vi "GetProgramName.vi"(8 "error in":errorcluster, 11 "VISA resource name":refnum<visa-resource-name>) -> (0 "error out":errorcluster, 2 "Currently loaded program name response":string, 3 "VISA resource name out":refnum<visa-resource-name>)   [LabVIEW 2023, in "Thermotron 8800.lvlib"]
doc: "PNAM\nCommand name: Send program name\nCommand type: Program status\nDescription: Queries the 8800 for the name of the currently loaded program. The 8800 responds with the program’s assigned name (a string up to 15 characters long). If there is no currently loaded program name available, the 8800 will respond with “Untitled”.\nSyntax: PNAM?\nData type: String\nQuery example 1: PNAM?\n8800 response: STRESS SCREEN40 (The name of the currently loaded program is STRESS SCREEN40.)\nQuery example 2: PNAM?\n8800 response: Untitled (There is no currently loaded program name available.)"
uses:
  Thermotron 8800.lvlib
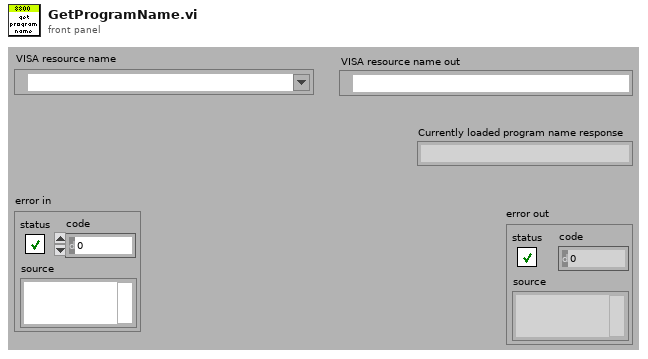
[diagram p1: front panel]
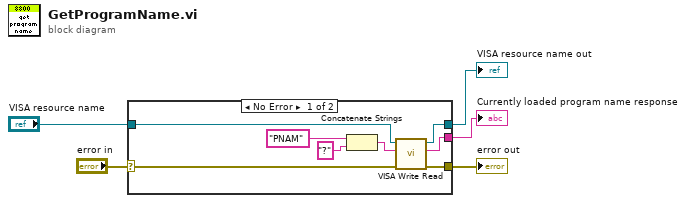
[diagram p0: block diagram]
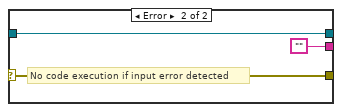
[diagram p2: hidden frame]
diagram:
  n1 = case shown="No Error" "error in" {
    selector: "error in" -> [w11 w16]
    tunnel: [w10 w16] -> w4
    tunnel: "VISA resource name" -> [w9 w15]
    tunnel: [w8 w15] -> w2
    tunnel: [w7 ""] -> w1
    frame No Error {
      n2 = Concatenate Strings("PNAM" ("string"), "?" ("string")) -> (w12:string)
      n3 = call "VISA Write Read.vi"("error in (no error)"=w11, "8800 Command"=w12, "VISA Refnum in"=w9) -> ("error out"=w10:errorcluster, "read buffer"=w7:string, "VISA Refnum out"=w8:refnum<visa-resource-name>)  [unwired: 6 in]
    }
    frame Error {
      # "No code execution if input error detected"
    }
  }
  "error out" <- w4
  "VISA resource name out" <- w2
  "Currently loaded program name response" <- w1
